vi "GRBL_Write .vi"(8 "error in":errorcluster, 10 "GRBL Cmd":string[](array[string])=["G10P0L20X0Y0", "G90", "G00X40", "G00Y80", "G00X0Y0", "M30"], 11 "VISA resource name":refnum<visa-resource-name>) -> (0 "error out":errorcluster, 3 "VISA resource name out":refnum<visa-resource-name>)   [LabVIEW 2014, in "QwaveSys Raspberry Pi Library.lvlib"]
uses:
  QwaveSys Raspberry Pi Library.lvlib
panel:
  out "return count 2":u32
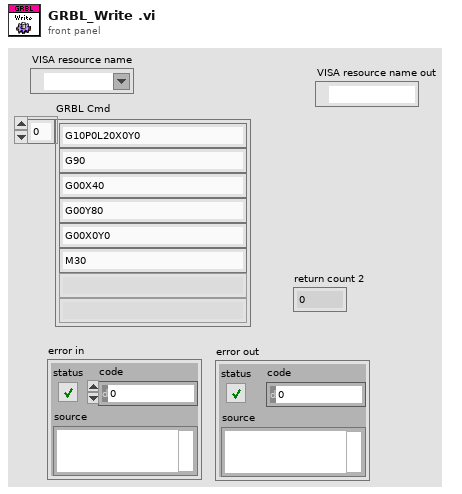
[diagram p1: front panel]
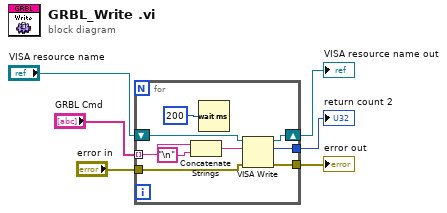
[diagram p0: block diagram]
diagram:
  n1 = for {
    tunnel: [w15] -> w6
    shift-right: [w13] -> w4
    shift-left: "VISA resource name" -> [w14]
    tunnel: [w12] -> w2
    tunnel: "error in" -> [w11]
    tunnel: "GRBL Cmd" -> [w9] mode=indexing
    n2 = Concatenate Strings(w9, "\n" ("Line Feed Constant")) -> (w7:string)
    n3 = Wait (ms)(milliseconds to wait=u32 200) -> ()  [unwired: 1 out]
    n4 = VISA Write(VISA resource name=w14, write buffer=w7, error in (no error)=w11) -> (VISA resource name out=w13:refnum<visa-resource-name>, return count=w15:u32, error out=w12:errorcluster)
  }
  "error out" <- w2
  "return count 2" <- w6
  "VISA resource name out" <- w4
